vi "screen for manual mode operation.vi"() -> ()   [LabVIEW 2025]
uses:
  <vilib>/picture/picture.llb/Draw True-Color Pixmap.vi
panel:
  out "?":picture
  out "?":picture
  in  "Rotation Angle (degree) 2":dbl(knob) scale=-180.0..180.0
  in  "Scale 2":dbl(slide)=1.0 scale=0.1..10.0
  in  "stop 3":bool
  in  "Rotation Angle (degree)":dbl(knob) scale=-180.0..180.0
  in  "Scale":dbl(slide)=1.0 scale=0.1..10.0
  in  "stop 2":bool
  out "?":string="Job Name"
  out "?":timestamp=timestamp(3840529035.531137 s since 1904-01-01) format="%<%d %b %Y | %H:%M>T"
  out "?":timestamp=timestamp(3840529035.531137 s since 1904-01-01) format="%<%Hh %Mm %Ss>T"
  in  "?":bool
  in  "RIGHT":bool
  in  "LEFT":bool
  in  "DOWN":bool
  in  "stop":bool
  in  "UP":bool
  # "Y Axis"
  # "X Axis"
  # "Manual Mode"
  # "JOB STARTED ON"
  # "Time since start"
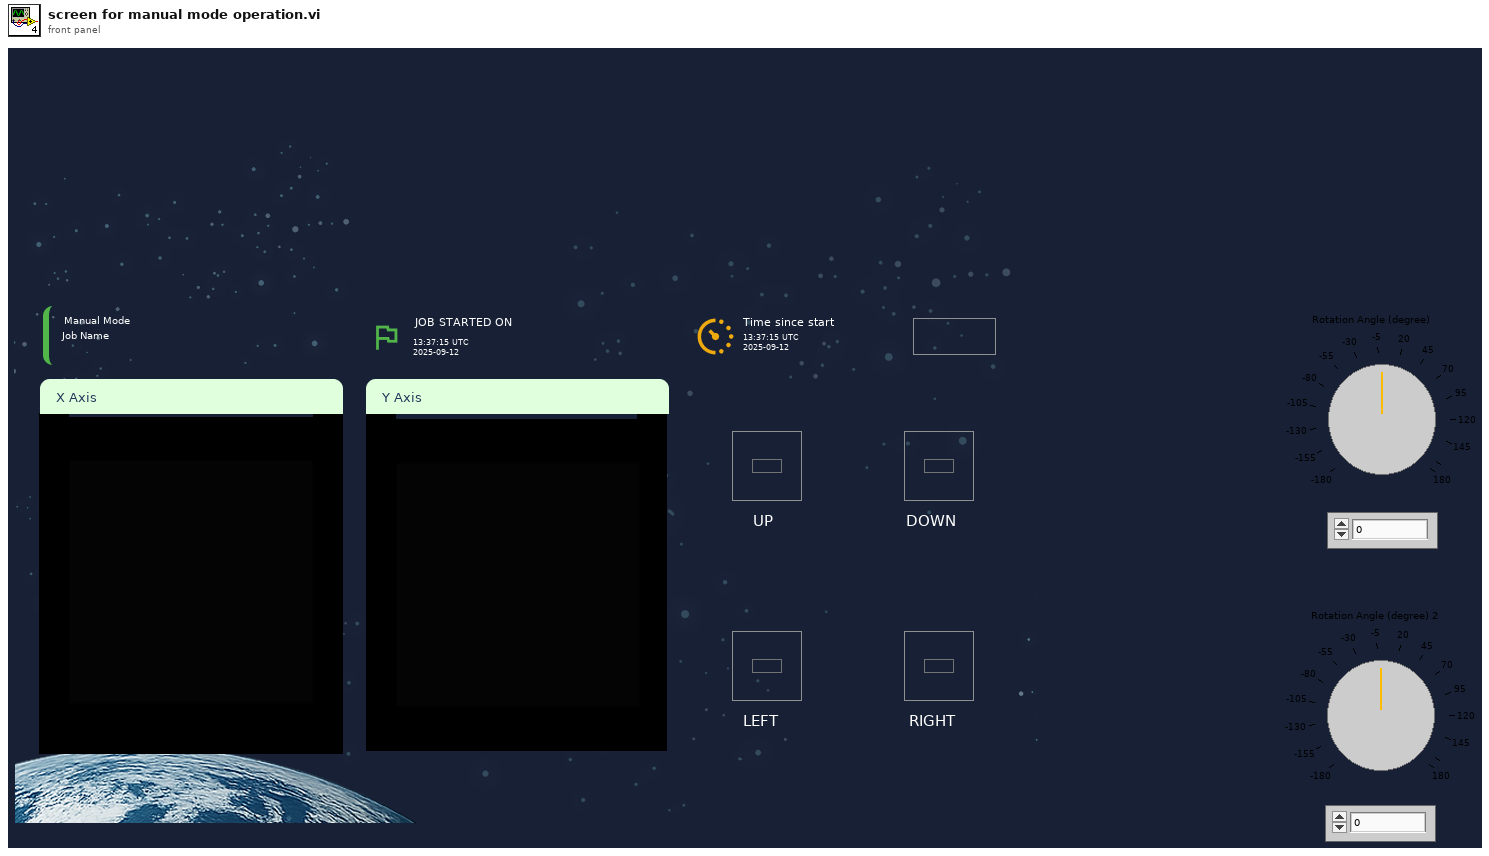
[diagram p1: front panel]
types:
  T1 = typedef "imagedata.ctl" = cluster{"image type":i32, "image depth":i32, "image":u8[], "mask":u8[], "colors":u32[], "Rectangle":cluster{"left":i16, "top":i16, "right":i16, "bottom":i16}}
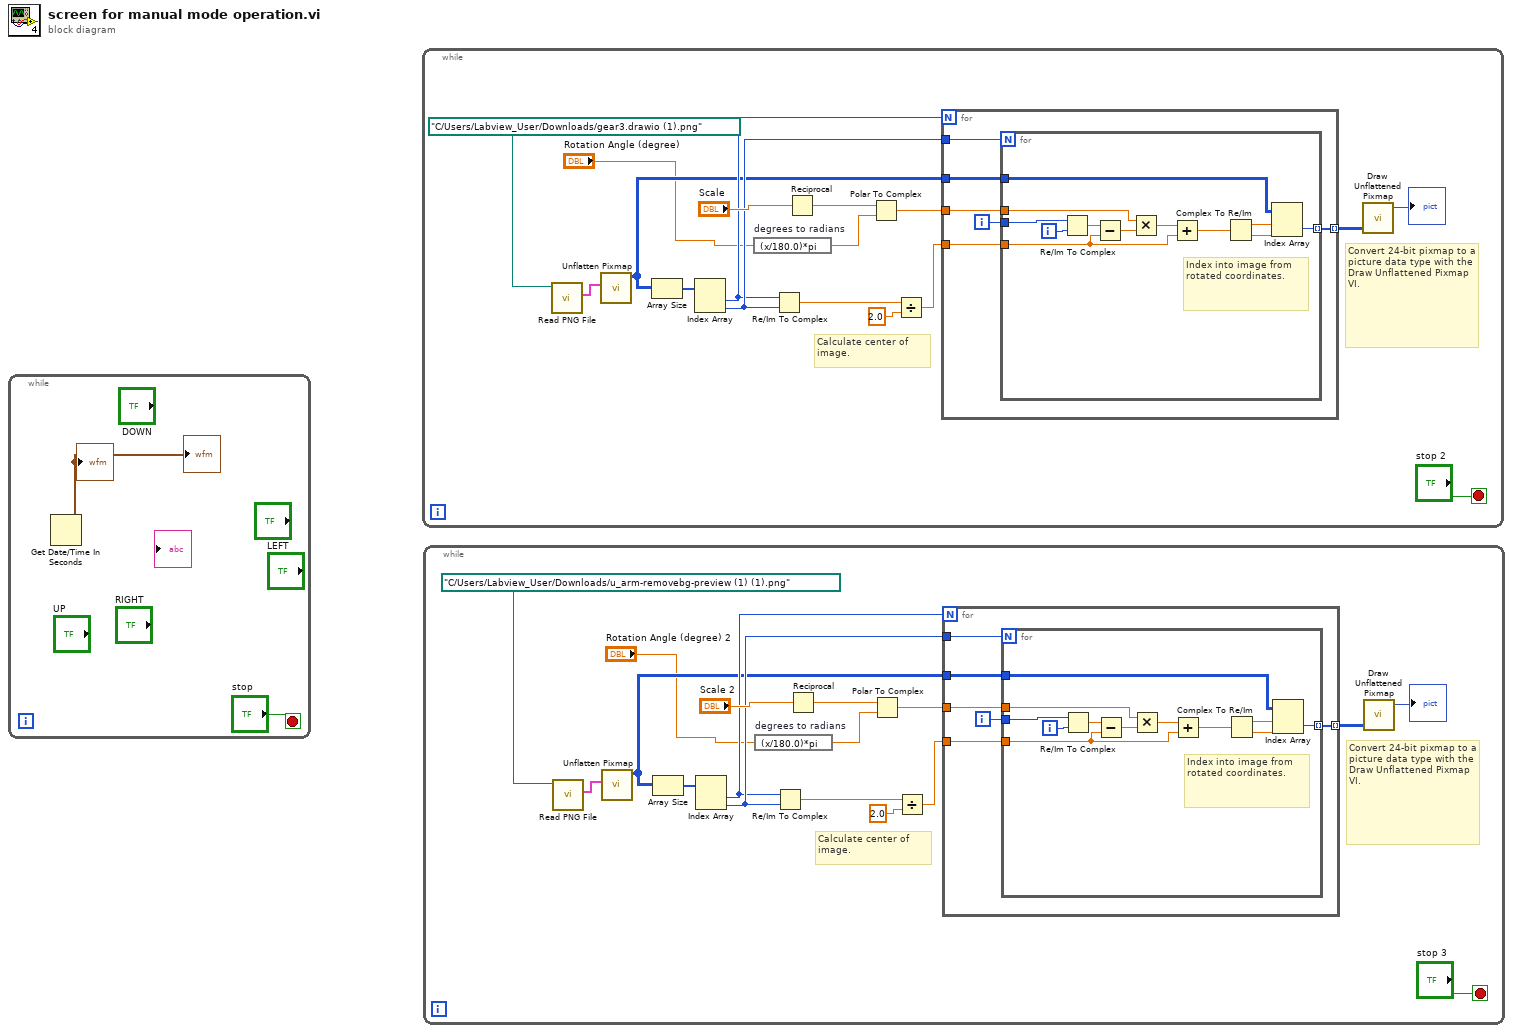
[diagram p0: block diagram]
diagram:
  n1 = while {
    stop <- "stop" stop-if-true
    n2 = Get Date/Time In Seconds() -> (seconds since 1Jan1904=→"?" →"?":timestamp)
  }
  n3 = while {
    stop <- "stop 2" stop-if-true
    # "Calculate center of image."
    # "Convert 24-bit pixmap to a picture data type with the Draw Unflattened Pixmap VI."
    n4 = call <vilib>:"Read PNG File.vi"("path to PNG file"=path "C:/Users/Labview_User/Downloads/gear3.drawio (1).png") -> ("image data"=w7:T1)  [unwired: 8 in, 2 out]
    n5 = call <vilib>:"Unflatten Pixmap.vi"("image data"=w7) -> ("24-bit pixmap"=w8:u32[][])  [unwired: 4 in, 6 out]
    n6 = Array Size(array=w8) -> (size(s)=w13:i32[])
    n7 = Index Array(array=w13) -> (element #1=w11:i32, element #2=w12:i32)  [unwired: 2 in]
    n8 = expression code="(x/180.0)*pi" "degrees to radians"("Rotation Angle (degree)") -> (w6:dbl)
    n9 = Re/Im To Complex(1:w12, 2:w11) -> (0:w14:cdb)
    n10 = Reciprocal(x="Scale") -> (1/x=w16:dbl)
    n11 = Polar To Complex(1:w6, 2:w16) -> (0:w15:cdb)
    n12 = Divide(x=w14, y=2.0) -> (x/y=w10:cdb)
    n13 = for {
      N: w11 -> [_]
      tunnel: w12 -> [w24]
      tunnel: w8 -> [w23]
      tunnel: [w22] -> w18 mode=indexing
      tunnel: w15 -> [w21]
      tunnel: w10 -> [w20]
      i -> [w25]
      n14 = for {
        N: w24 -> [_]
        tunnel: w25 -> [w34]
        tunnel: w23 -> [w37]
        tunnel: [w36] -> w22 mode=indexing
        tunnel: w21 -> [w27]
        tunnel: w20 -> [w26]
        i -> [w35]
        # "Index into image from rotated coordinates."
        n15 = Re/Im To Complex(1:w35, 2:w34) -> (0:w33:cdb)
        n16 = Subtract(x=w33, y=w26) -> (x-y=w32:cdb)
        n17 = Multiply(x=w27, y=w32) -> (x*y=w31:cdb)
        n18 = Add(x=w31, y=w26) -> (x+y=w30:cdb)
        n19 = Complex To Re/Im(x + iy=w30) -> (x=w29:dbl, y=w28:dbl)
        n20 = Index Array(array=w37, index (row)=w29, index (col)=w28) -> (element=w36:u32)
      }
    }
    n21 = call-poly <vilib>:"Draw Unflattened Pixmap.vi"("data (RGB format)"=w18) -> ("new picture"=→"?":picture)  [unwired: 8 in]
  }
  n22 = while {
    stop <- "stop 3" stop-if-true
    # "Calculate center of image."
    # "Convert 24-bit pixmap to a picture data type with the Draw Unflattened Pixmap VI."
    n23 = call <vilib>:"Read PNG File.vi"("path to PNG file"=path "C:/Users/Labview_User/Downloads/u_arm-removebg-preview (1) (1).png" ("path to PNG file 2")) -> ("image data"=w42:T1)  [unwired: 8 in, 2 out]
    n24 = call <vilib>:"Unflatten Pixmap.vi"("image data"=w42) -> ("24-bit pixmap"=w43:u32[][])  [unwired: 4 in, 6 out]
    n25 = Array Size(array=w43) -> (size(s)=w48:i32[])
    n26 = Index Array(array=w48) -> (element #1=w46:i32, element #2=w47:i32)  [unwired: 2 in]
    n27 = expression code="(x/180.0)*pi" "degrees to radians"("Rotation Angle (degree) 2") -> (w41:dbl)
    n28 = Re/Im To Complex(1:w47, 2:w46) -> (0:w49:cdb)
    n29 = Reciprocal(x="Scale 2") -> (1/x=w51:dbl)
    n30 = Polar To Complex(1:w41, 2:w51) -> (0:w50:cdb)
    n31 = Divide(x=w49, y=2.0) -> (x/y=w45:cdb)
    n32 = for {
      N: w46 -> [_]
      tunnel: w47 -> [w59]
      tunnel: w43 -> [w58]
      tunnel: [w57] -> w53 mode=indexing
      tunnel: w50 -> [w56]
      tunnel: w45 -> [w55]
      i -> [w60]
      n33 = for {
        N: w59 -> [_]
        tunnel: w60 -> [w69]
        tunnel: w58 -> [w72]
        tunnel: [w71] -> w57 mode=indexing
        tunnel: w56 -> [w62]
        tunnel: w55 -> [w61]
        i -> [w70]
        # "Index into image from rotated coordinates."
        n34 = Re/Im To Complex(1:w70, 2:w69) -> (0:w68:cdb)
        n35 = Subtract(x=w68, y=w61) -> (x-y=w67:cdb)
        n36 = Multiply(x=w62, y=w67) -> (x*y=w66:cdb)
        n37 = Add(x=w66, y=w61) -> (x+y=w65:cdb)
        n38 = Complex To Re/Im(x + iy=w65) -> (x=w64:dbl, y=w63:dbl)
        n39 = Index Array(array=w72, index (row)=w64, index (col)=w63) -> (element=w71:u32)
      }
    }
    n40 = call-poly <vilib>:"Draw Unflattened Pixmap.vi"("data (RGB format)"=w53) -> ("new picture"=→"?":picture)  [unwired: 8 in]
  }
